vi "Digital Configure Port.vi"(8 "Error In":errorcluster, 10 "DIO Pins":u8[](array[numeric]), 11 "ChipKit Resource":T1={"COM Port"="", "Board Type"=enum."ChipKit uC32", "Connection Type"=enum."USB / Serial", "Baud Rate (115200)"=15, "Bytes Per Packet (15)"=15}) -> (0 "Error Out":errorcluster, 3 "ChipKit Resource":T1={"COM Port"="", "Board Type"=enum."ChipKit uC32", "Connection Type"=enum."USB / Serial", "Baud Rate (115200)"=15, "Bytes Per Packet (15)"=15})   [LabVIEW 2011, in "LabVIEW Interface for ChipKit.lvlib"]
uses:
  LabVIEW Interface for ChipKit.lvlib
  Private/Type Defs/Chipkit Resource.ctl
  Private/Type Defs/Board Type.ctl
  Private/Type Defs/Connection Type.ctl
  Private/Type Defs/Command.ctl
panel:
  out "Read Buffer":string
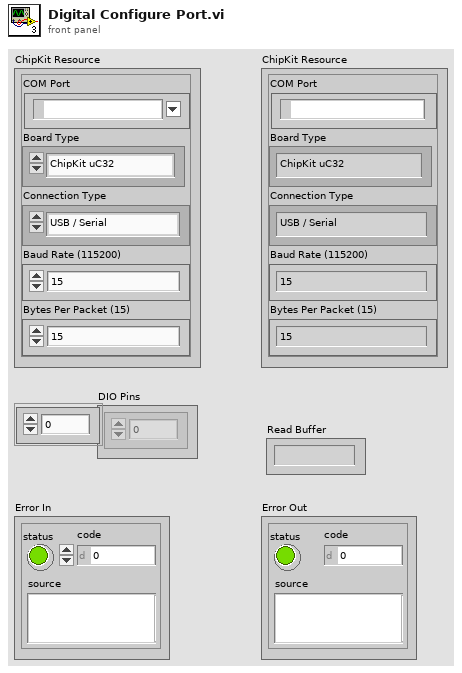
[diagram p1: front panel]
types:
  T1 = typedef "LabVIEW Interface for ChipKit.lvlib/Chipkit Resource.ctl" = cluster{"COM Port":refnum<visa-resource-name>, "Board Type":T2, "Connection Type":T3, "Baud Rate (115200)":u32, "Bytes Per Packet (15)":u32}
  T2 = typedef "LabVIEW Interface for ChipKit.lvlib/Board Type.ctl" = enum16{"ChipKit uC32", "ChipKit Uno32", "ChipKit Max32"}
  T3 = typedef "LabVIEW Interface for ChipKit.lvlib/Connection Type.ctl" = enum8{"USB / Serial", "XBEE", "BlueSmirf (Bluetooth)"}
  T4 = typedef "LabVIEW Interface for ChipKit.lvlib/Command.ctl" = enum8{"setArduinoMode", "flushSerial", "setPinMode", "digitalWritePin", "digitalWritePort", "tone", "digitalReadPin", "digitalReadPort", "analogReadPin", "analogReadPort", "pwmWritePin", "pwmWritePort", "sevenSegment_Configure", "sevenSegment_Write", "I2C Init", "I2C Write", "I2C Read", "SPI Init", "SPI Set Bit Order", "SPI Set Clock Divider", "SPI Set Data Mode", "SPI Send / Receive", "SPI Close", "Servo Set Num Servos", "Servo Config Servo", "Servo Write Angle", "Servo Read Angle", "Servo Write Pulse Width", "Servo Read Pulse Width", "Servo Detach", "LCD Init", "LCD Set Size", "LCD Set Cursor Mode", "LCD Clear", "LCD Set Cursor Position", "LCD Print", "LCD Display Power", "LCD Scroll Display", "LCD Autoscroll", "LCD Print Direction", "LCD Create Custom Char", "LCD Print Custom Char", "contAcqOn", "contAcqOff", "getFirmwareVersion", "FiniteSampleStart", "NA", "NA2", "Configure Stepper", "Stepper Write", "Stepper Detach", "Stepper Steps To Go", "Configure Digital Port"}
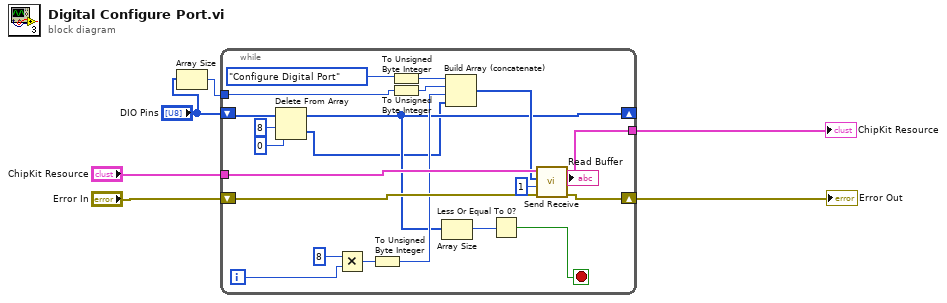
[diagram p0: block diagram]
diagram:
  n1 = Array Size(array="DIO Pins") -> (size(s)=w1:i32)
  n2 = while {
    tunnel: "ChipKit Resource" -> [w28]
    tunnel: [w26] -> w4
    shift-right: [w24] -> w3
    shift-left: "Error In" -> [w27]
    shift-right: [w11] -> _
    shift-left: "DIO Pins" -> [w23]
    tunnel: w1 -> [w16]
    i -> [w14]
    stop <- w9 stop-if-true
    n3 = Delete From Array(array=w23, length=8, index=0) -> (deleted portion=w8:u8[], array with subset deleted=w11:u8[])
    n4 = Multiply(x=8, y=w14) -> (x*y=w15:i32)
    n5 = To Unsigned Byte Integer(number=w15) -> (unsigned 8bit integer=w12:u8)
    n6 = To Unsigned Byte Integer(number=Command."Configure Digital Port" ("Command")) -> (unsigned 8bit integer=w20:u8)
    n7 = To Unsigned Byte Integer(number=w16) -> (unsigned 8bit integer=w17:u8)
    n8 = Array Size(array=w11) -> (size(s)=w10:i32)
    n9 = Build Array (concatenate)(w20, w17, w12, w8) -> (w18:u8[])
    n10 = Less Or Equal To 0?(x=w10) -> (x <= 0?=w9:bool)
    n11 = call "Send Receive.vi"("Error In"=w27, "Bytes To Read (0)"=u8 1, "Data"=w18, "ChipKit Resource"=w28) -> ("Error Out"=w24:errorcluster, "Read Buffer"=→"Read Buffer":string, "ChipKit Resource"=w26:T1)  [unwired: 5 in]
  }
  "Error Out" <- w3
  "ChipKit Resource" <- w4
